vi "App - analyze RUS V6.vi"() -> ()   [LabVIEW 2021] (continued)
 "temperature str"="14.44900", "file path"=path "D:/Data/Ultrasound/LSCO/LSCO22__130814c/5_Cooling_2nd_try/September_2014/091814/14.44900K_500_2500_2.10000V_0.00000T_Sep18-2014__02-05-45_001_091814.bin", "last mod"=timestamp(3493865145 s since 1904-01-01), "file name str"="D:\\Data\\Ultrasound\\LSCO\\LSCO22__130814c\\5_Cooling_2nd_try\\September_2014\\091814\\14.44900K_500_2500_2.10000V_0.00000T_Sep18-2014__02-05-45_001_091814.bin", "mod time(min)"=58231085.75, "file format"=enum."binary", "power(V)"=2.1, "Magn Field(T) "=0.0}, {"temperature"=14.445, "temperature str"="14.44500", "file path"=path "D:/Data/Ultrasound/LSCO/LSCO22__130814c/5_Cooling_2nd_try/September_2014/091814/14.44500K_500_2500_2.10000V_0.00000T_Sep18-2014__02-07-04_001_091814.bin", "last mod"=timestamp(3493865224 s since 1904-01-01), "file name str"="D:\\Data\\Ultrasound\\LSCO\\LSCO22__130814c\\5_Cooling_2nd_try\\September_2014\\091814\\14.44500K_500_2500_2.10000V_0.00000T_Sep18-2014__02-07-04_001_091814.bin", "mod time(min)"=58231087.06666667, "file format"=enum."binary", "power(V)"=2.1, "Magn Field(T) "=0.0}, {"temperature"=14.447, "temperature str"="14.44700", "file path"=path "D:/Data/Ultrasound/LSCO/LSCO22__130814c/5_Cooling_2nd_try/September_2014/091814/14.44700K_500_2500_2.10000V_0.00000T_Sep18-2014__02-08-23_001_091814.bin", "last mod"=timestamp(3493865303 s since 1904-01-01), "file name str"="D:\\Data\\Ultrasound\\LSCO\\LSCO22__130814c\\5_Cooling_2nd_try\\September_2014\\091814\\14.44700K_500_2500_2.10000V_0.00000T_Sep18-2014__02-08-23_001_091814.bin", "mod time(min)"=58231088.38333333, "file format"=enum."binary", "power(V)"=2.1, "Magn Field(T) "=0.0}, {"temperature"=14.443, "temperature str"="14.44300", "file path"=path "D:/Data/Ultrasound/LSCO/LSCO22__130814c/5_Cooling_2nd_try/September_2014/091814/14.44300K_500_2500_2.10000V_0.00000T_Sep18-2014__02-09-43_001_091814.bin", "last mod"=timestamp(3493865383 s since 1904-01-01), "file name str"="D:\\Data\\Ultrasound\\LSCO\\LSCO22__130814c\\5_Cooling_2nd_try\\September_2014\\091814\\14.44300K_500_2500_2.10000V_0.00000T_Sep18-2014__02-09-43_001_091814.bin", "mod time(min)"=58231089.71666667, "file format"=enum."binary", "power(V)"=2.1, "Magn Field(T) "=0.0}, {"temperature"=14.439, "temperature str"="14.43900", "file path"=path "D:/Data/Ultrasound/LSCO/LSCO22__130814c/5_Cooling_2nd_try/September_2014/091814/14.43900K_500_2500_2.10000V_0.00000T_Sep18-2014__02-11-02_001_091814.bin", "last mod"=timestamp(3493865462 s since 1904-01-01), "file name str"="D:\\Data\\Ultrasound\\LSCO\\LSCO22__130814c\\5_Cooling_2nd_try\\September_2014\\091814\\14.43900K_500_2500_2.10000V_0.00000T_Sep18-2014__02-11-02_001_091814.bin", "mod time(min)"=58231091.03333333, "file format"=enum."binary", "power(V)"=2.1, "Magn Field(T) "=0.0}, {"temperature"=14.439, "temperature str"="14.43900", "file path"=path "D:/Data/Ultrasound/LSCO/LSCO22__130814c/5_Cooling_2nd_try/September_2014/091814/14.43900K_500_2500_2.10000V_0.00000T_Sep18-2014__02-12-21_001_091814.bin", "last mod"=timestamp(3493865541 s since 1904-01-01), "file name str"="D:\\Data\\Ultrasound\\LSCO\\LSCO22__130814c\\5_Cooling_2nd_try\\September_2014\\091814\\14.43900K_500_2500_2.10000V_0.00000T_Sep18-2014__02-12-21_001_091814.bin", "mod time(min)"=58231092.35, "file format"=enum."binary", "power(V)"=2.1, "Magn Field(T) "=0.0}, {"temperature"=14.439, "temperature str"="14.43900", "file path"=path "D:/Data/Ultrasound/LSCO/LSCO22__130814c/5_Cooling_2nd_try/September_2014/091814/14.43900K_500_2500_2.10000V_0.00000T_Sep18-2014__02-13-41_001_091814.bin", "last mod"=timestamp(3493865621 s since 1904-01-01), "file name str"="D:\\Data\\Ultrasound\\LSCO\\LSCO22__130814c\\5_Cooling_2nd_try\\September_2014\\091814\\14.43900K_500_2500_2.10000V_0.00000T_Sep18-2014__02-13-41_001_091814.bin", "mod time(min)"=58231093.68333333, "file format"=enum."binary", "power(V)"=2.1, "Magn Field(T) "=0.0}, {"temperature"=14.439, "temperature str"="14.43900", "file path"=path "D:/Data/Ultrasound/LSCO/LSCO22__130814c/5_Cooling_2nd_try/September_2014/091814/14.43900K_500_2500_2.10000V_0.00000T_Sep18-2014__02-15-00_001_091814.bin", "last mod"=timestamp(3493865700 s since 1904-01-01), "file name str"="D:\\Data\\Ultrasound\\LSCO\\LSCO22__130814c\\5_Cooling_2nd_try\\September_2014\\091814\\14.43900K_500_2500_2.10000V_0.00000T_Sep18-2014__02-15-00_001_091814.bin", "mod time(min)"=58231095.0, "file format"=enum."binary", "power(V)"=2.1, "Magn Field(T) "=0.0}, {"temperature"=14.44, "temperature str"="14.44000", "file path"=path "D:/Data/Ultrasound/LSCO/LSCO22__130814c/5_Cooling_2nd_try/September_2014/091814/14.44000K_500_2500_2.10000V_0.00000T_Sep18-2014__02-16-20_001_091814.bin", "last mod"=timestamp(3493865780 s since 1904-01-01), "file name str"="D:\\Data\\Ultrasound\\LSCO\\LSCO22__130814c\\5_Cooling_2nd_try\\September_2014\\091814\\14.44000K_500_2500_2.10000V_0.00000T_Sep18-2014__02-16-20_001_091814.bin", "mod time(min)"=58231096.333333336, "file format"=enum."binary", "power(V)"=2.1, "Magn Field(T) "=0.0}, {"temperature"=14.433, "temperature str"="14.43300", "file path"=path "D:/Data/Ultrasound/LSCO/LSCO22__130814c/5_Cooling_2nd_try/September_2014/091814/14.43300K_500_2500_2.10000V_0.00000T_Sep18-2014__02-17-39_001_091814.bin", "last mod"=timestamp(3493865859 s since 1904-01-01), "file name str"="D:\\Data\\Ultrasound\\LSCO\\LSCO22__130814c\\5_Cooling_2nd_try\\September_2014\\091814\\14.43300K_500_2500_2.10000V_0.00000T_Sep18-2014__02-17-39_001_091814.bin", "mod time(min)"=58231097.65, "file format"=enum."binary", "power(V)"=2.1, "Magn Field(T) "=0.0}, {"temperature"=14.434, "temperature str"="14.43400", "file path"=path "D:/Data/Ultrasound/LSCO/LSCO22__130814c/5_Cooling_2nd_try/September_2014/091814/14.43400K_500_2500_2.10000V_0.00000T_Sep18-2014__02-18-58_001_091814.bin", "last mod"=timestamp(3493865938 s since 1904-01-01), "file name str"="D:\\Data\\Ultrasound\\LSCO\\LSCO22__130814c\\5_Cooling_2nd_try\\September_2014\\091814\\14.43400K_500_2500_2.10000V_0.00000T_Sep18-2014__02-18-58_001_091814.bin", "mod time(min)"=58231098.96666667, "file format"=enum."binary", "power(V)"=2.1, "Magn Field(T) "=0.0}, {"temperature"=14.43, "temperature str"="14.43000", "file path"=path "D:/Data/Ultrasound/LSCO/LSCO22__130814c/5_Cooling_2nd_try/September_2014/091814/14.43000K_500_2500_2.10000V_0.00000T_Sep18-2014__02-20-18_001_091814.bin", "last mod"=timestamp(3493866018 s since 1904-01-01), "file name str"="D:\\Data\\Ultrasound\\LSCO\\LSCO22__130814c\\5_Cooling_2nd_try\\September_2014\\091814\\14.43000K_500_2500_2.10000V_0.00000T_Sep18-2014__02-20-18_001_091814.bin", "mod time(min)"=58231100.3, "file format"=enum."binary", "power(V)"=2.1, "Magn Field(T) "=0.0}, {"temperature"=14.43, "temperature str"="14.43000", "file path"=path "D:/Data/Ultrasound/LSCO/LSCO22__130814c/5_Cooling_2nd_try/September_2014/091814/14.43000K_500_2500_2.10000V_0.00000T_Sep18-2014__02-21-37_001_091814.bin", "last mod"=timestamp(3493866097 s since 1904-01-01), "file name str"="D:\\Data\\Ultrasound\\LSCO\\LSCO22__130814c\\5_Cooling_2nd_try\\September_2014\\091814\\14.43000K_500_2500_2.10000V_0.00000T_Sep18-2014__02-21-37_001_091814.bin", "mod time(min)"=58231101.61666667, "file format"=enum."binary", "power(V)"=2.1, "Magn Field(T) "=0.0}, {"temperature"=14.43, "temperature str"="14.43000", "file path"=path "D:/Data/Ultrasound/LSCO/LSCO22__130814c/5_Cooling_2nd_try/September_2014/091814/14.43000K_500_2500_2.10000V_0.00000T_Sep18-2014__02-22-57_001_091814.bin", "last mod"=timestamp(3493866177 s since 1904-01-01), "file name str"="D:\\Data\\Ultrasound\\LSCO\\LSCO22__130814c\\5_Cooling_2nd_try\\September_2014\\091814\\14.43000K_500_2500_2.10000V_0.00000T_Sep18-2014__02-22-57_001_091814.bin", "mod time(min)"=58231102.95, "file format"=enum."binary", "power(V)"=2.1, "Magn Field(T) "=0.0}, {"temperature"=14.434, "temperature str"="14.43400", "file path"=path "D:/Data/Ultrasound/LSCO/LSCO22__130814c/5_Cooling_2nd_try/September_2014/091814/14.43400K_500_2500_2.10000V_0.00000T_Sep18-2014__02-24-16_001_091814.bin", "last mod"=timestamp(3493866256 s since 1904-01-01), "file name str"="D:\\Data\\Ultrasound\\LSCO\\LSCO22__130814c\\5_Cooling_2nd_try\\September_2014\\091814\\14.43400K_500_2500_2.10000V_0.00000T_Sep18-2014__02-24-16_001_091814.bin", "mod time(min)"=58231104.266666666, "file format"=enum."binary", "power(V)"=2.1, "Magn Field(T) "=0.0}, {"temperature"=14.434, "temperature str"="14.43400", "file path"=path "D:/Data/Ultrasound/LSCO/LSCO22__130814c/5_Cooling_2nd_try/September_2014/091814/14.43400K_500_2500_2.10000V_0.00000T_Sep18-2014__02-25-35_001_091814.bin", "last mod"=timestamp(3493866335 s since 1904-01-01), "file name str"="D:\\Data\\Ultrasound\\LSCO\\LSCO22__130814c\\5_Cooling_2nd_try\\September_2014\\091814\\14.43400K_500_2500_2.10000V_0.00000T_Sep18-2014__02-25-35_001_091814.bin", "mod time(min)"=58231105.583333336, "file format"=enum."binary", "power(V)"=2.1, "Magn Field(T) "=0.0}, {"temperature"=14.431, "temperature str"="14.43100", "file path"=path "D:/Data/Ultrasound/LSCO/LSCO22__130814c/5_Cooling_2nd_try/September_2014/091814/14.43100K_500_2500_2.10000V_0.00000T_Sep18-2014__02-26-55_001_091814.bin", "last mod"=timestamp(3493866415 s since 1904-01-01), "file name str"="D:\\Data\\Ultrasound\\LSCO\\LSCO22__130814c\\5_Cooling_2nd_try\\September_2014\\091814\\14.43100K_500_2500_2.10000V_0.00000T_Sep18-2014__02-26-55_001_091814.bin", "mod time(min)"=58231106.916666664, "file format"=enum."binary", "power(V)"=2.1, "Magn Field(T) "=0.0}, {"temperature"=14.429, "temperature str"="14.42900", "file path"=path "D:/Data/Ultrasound/LSCO/LSCO22__130814c/5_Cooling_2nd_try/September_2014/091814/14.42900K_500_2500_2.10000V_0.00000T_Sep18-2014__02-28-14_001_091814.bin", "last mod"=timestamp(3493866494 s since 1904-01-01), "file name str"="D:\\Data\\Ultrasound\\LSCO\\LSCO22__130814c\\5_Cooling_2nd_try\\September_2014\\091814\\14.42900K_500_2500_2.10000V_0.00000T_Sep18-2014__02-28-14_001_091814.bin", "mod time(min)"=58231108.233333334, "file format"=enum."binary", "power(V)"=2.1, "Magn Field(T) "=0.0}, {"temperature"=14.426, "temperature str"="14.42600", "file path"=path "D:/Data/Ultrasound/LSCO/LSCO22__130814c/5_Cooling_2nd_try/September_2014/091814/14.42600K_500_2500_2.10000V_0.00000T_Sep18-2014__02-29-33_001_091814.bin", "last mod"=timestamp(3493866573 s since 1904-01-01), "file name str"="D:\\Data\\Ultrasound\\LSCO\\LSCO22__130814c\\5_Cooling_2nd_try\\September_2014\\091814\\14.42600K_500_2500_2.10000V_0.00000T_Sep18-2014__02-29-33_001_091814.bin", "mod time(min)"=58231109.55, "file format"=enum."binary", "power(V)"=2.1, "Magn Field(T) "=0.0}, {"temperature"=14.429, "temperature str"="14.42900", "file path"=path "D:/Data/Ultrasound/LSCO/LSCO22__130814c/5_Cooling_2nd_try/September_2014/091814/14.42900K_500_2500_2.10000V_0.00000T_Sep18-2014__02-30-53_001_091814.bin", "last mod"=timestamp(3493866653 s since 1904-01-01), "file name str"="D:\\Data\\Ultrasound\\LSCO\\LSCO22__130814c\\5_Cooling_2nd_try\\September_2014\\091814\\14.42900K_500_2500_2.10000V_0.00000T_Sep18-2014__02-30-53_001_091814.bin", "mod time(min)"=58231110.88333333, "file format"=enum."binary", "power(V)"=2.1, "Magn Field(T) "=0.0}, {"temperature"=14.429, "temperature str"="14.42900", "file path"=path "D:/Data/Ultrasound/LSCO/LSCO22__130814c/5_Cooling_2nd_try/September_2014/091814/14.42900K_500_2500_2.10000V_0.00000T_Sep18-2014__02-32-12_001_091814.bin", "last mod"=timestamp(3493866732 s since 1904-01-01), "file name str"="D:\\Data\\Ultrasound\\LSCO\\LSCO22__130814c\\5_Cooling_2nd_try\\September_2014\\091814\\14.42900K_500_2500_2.10000V_0.00000T_Sep18-2014__02-32-12_001_091814.bin", "mod time(min)"=58231112.2, "file format"=enum."binary", "power(V)"=2.1, "Magn Field(T) "=0.0}, {"temperature"=14.425, "temperature str"="14.42500", "file path"=path "D:/Data/Ultrasound/LSCO/LSCO22__130814c/5_Cooling_2nd_try/September_2014/091814/14.42500K_500_2500_2.10000V_0.00000T_Sep18-2014__02-33-32_001_091814.bin", "last mod"=timestamp(3493866812 s since 1904-01-01), "file name str"="D:\\Data\\Ultrasound\\LSCO\\LSCO22__130814c\\5_Cooling_2nd_try\\September_2014\\091814\\14.42500K_500_2500_2.10000V_0.00000T_Sep18-2014__02-33-32_001_091814.bin", "mod time(min)"=58231113.53333333, "file format"=enum."binary", "power(V)"=2.1, "Magn Field(T) "=0.0}, {"temperature"=14.426, "temperature str"="14.42600", "file path"=path "D:/Data/Ultrasound/LSCO/LSCO22__130814c/5_Cooling_2nd_try/September_2014/091814/14.42600K_500_2500_2.10000V_0.00000T_Sep18-2014__02-34-51_001_091814.bin", "last mod"=timestamp(3493866891 s since 1904-01-01), "file name str"="D:\\Data\\Ultrasound\\LSCO\\LSCO22__130814c\\5_Cooling_2nd_try\\September_2014\\091814\\14.42600K_500_2500_2.10000V_0.00000T_Sep18-2014__02-34-51_001_091814.bin", "mod time(min)"=58231114.85, "file format"=enum."binary", "power(V)"=2.1, "Magn Field(T) "=0.0}, {"temperature"=14.422, "temperature str"="14.42200", "file path"=path "D:/Data/Ultrasound/LSCO/LSCO22__130814c/5_Cooling_2nd_try/September_2014/091814/14.42200K_500_2500_2.10000V_0.00000T_Sep18-2014__02-36-10_001_091814.bin", "last mod"=timestamp(3493866970 s since 1904-01-01), "file name str"="D:\\Data\\Ultrasound\\LSCO\\LSCO22__130814c\\5_Cooling_2nd_try\\September_2014\\091814\\14.42200K_500_2500_2.10000V_0.00000T_Sep18-2014__02-36-10_001_091814.bin", "mod time(min)"=58231116.166666664, "file format"=enum."binary", "power(V)"=2.1, "Magn Field(T) "=0.0}, {"temperature"=14.424, "temperature str"="14.42400", "file path"=path "D:/Data/Ultrasound/LSCO/LSCO22__130814c/5_Cooling_2nd_try/September_2014/091814/14.42400K_500_2500_2.10000V_0.00000T_Sep18-2014__02-37-30_001_091814.bin", "last mod"=timestamp(3493867050 s since 1904-01-01), "file name str"="D:\\Data\\Ultrasound\\LSCO\\LSCO22__130814c\\5_Cooling_2nd_try\\September_2014\\091814\\14.42400K_500_2500_2.10000V_0.00000T_Sep18-2014__02-37-30_001_091814.bin", "mod time(min)"=58231117.5, "file format"=enum."binary", "power(V)"=2.1, "Magn Field(T) "=0.0}, {"temperature"=14.421, "temperature str"="14.42100", "file path"=path "D:/Data/Ultrasound/LSCO/LSCO22__130814c/5_Cooling_2nd_try/September_2014/091814/14.42100K_500_2500_2.10000V_0.00000T_Sep18-2014__02-38-49_001_091814.bin", "last mod"=timestamp(3493867129 s since 1904-01-01), "file name str"="D:\\Data\\Ultrasound\\LSCO\\LSCO22__130814c\\5_Cooling_2nd_try\\September_2014\\091814\\14.42100K_500_2500_2.10000V_0.00000T_Sep18-2014__02-38-49_001_091814.bin", "mod time(min)"=58231118.81666667, "file format"=enum."binary", "power(V)"=2.1, "Magn Field(T) "=0.0}, {"temperature"=14.418, "temperature str"="14.41800", "file path"=path "D:/Data/Ultrasound/LSCO/LSCO22__130814c/5_Cooling_2nd_try/September_2014/091814/14.41800K_500_2500_2.10000V_0.00000T_Sep18-2014__02-40-08_001_091814.bin", "last mod"=timestamp(3493867208 s since 1904-01-01), "file name str"="D:\\Data\\Ultrasound\\LSCO\\LSCO22__130814c\\5_Cooling_2nd_try\\September_2014\\091814\\14.41800K_500_2500_2.10000V_0.00000T_Sep18-2014__02-40-08_001_091814.bin", "mod time(min)"=58231120.13333333, "file format"=enum."binary", "power(V)"=2.1, "Magn Field(T) "=0.0}, {"temperature"=14.417, "temperature str"="14.41700", "file path"=path "D:/Data/Ultrasound/LSCO/LSCO22__130814c/5_Cooling_2nd_try/September_2014/091814/14.41700K_500_2500_2.10000V_0.00000T_Sep18-2014__02-41-28_001_091814.bin", "last mod"=timestamp(3493867288 s since 1904-01-01), "file name str"="D:\\Data\\Ultrasound\\LSCO\\LSCO22__130814c\\5_Cooling_2nd_try\\September_2014\\091814\\14.41700K_500_2500_2.10000V_0.00000T_Sep18-2014__02-41-28_001_091814.bin", "mod time(min)"=58231121.46666667, "file format"=enum."binary", "power(V)"=2.1, "Magn Field(T) "=0.0}, {"temperature"=14.415, "temperature str"="14.41500", "file path"=path "D:/Data/Ultrasound/LSCO/LSCO22__130814c/5_Cooling_2nd_try/September_2014/091814/14.41500K_500_2500_2.10000V_0.00000T_Sep18-2014__02-42-47_001_091814.bin", "last mod"=timestamp(3493867367 s since 1904-01-01), "file name str"="D:\\Data\\Ultrasound\\LSCO\\LSCO22__130814c\\5_Cooling_2nd_try\\September_2014\\091814\\14.41500K_500_2500_2.10000V_0.00000T_Sep18-2014__02-42-47_001_091814.bin", "mod time(min)"=58231122.78333333, "file format"=enum."binary", "power(V)"=2.1, "Magn Field(T) "=0.0}, {"temperature"=14.413, "temperature str"="14.41300", "file path"=path "D:/Data/Ultrasound/LSCO/LSCO22__130814c/5_Cooling_2nd_try/September_2014/091814/14.41300K_500_2500_2.10000V_0.00000T_Sep18-2014__02-44-07_001_091814.bin", "last mod"=timestamp(3493867447 s since 1904-01-01), "file name str"="D:\\Data\\Ultrasound\\LSCO\\LSCO22__130814c\\5_Cooling_2nd_try\\September_2014\\091814\\14.41300K_500_2500_2.10000V_0.00000T_Sep18-2014__02-44-07_001_091814.bin", "mod time(min)"=58231124.11666667, "file format"=enum."binary", "power(V)"=2.1, "Magn Field(T) "=0.0}, {"temperature"=14.414, "temperature str"="14.41400", "file path"=path "D:/Data/Ultrasound/LSCO/LSCO22__130814c/5_Cooling_2nd_try/September_2014/091814/14.41400K_500_2500_2.10000V_0.00000T_Sep18-2014__02-45-26_001_091814.bin", "last mod"=timestamp(3493867526 s since 1904-01-01), "file name str"="D:\\Data\\Ultrasound\\LSCO\\LSCO22__130814c\\5_Cooling_2nd_try\\September_2014\\091814\\14.41400K_500_2500_2.10000V_0.00000T_Sep18-2014__02-45-26_001_091814.bin", "mod time(min)"=58231125.43333333, "file format"=enum."binary", "power(V)"=2.1, "Magn Field(T) "=0.0}, {"temperature"=14.412, "temperature str"="14.41200", "file path"=path "D:/Data/Ultrasound/LSCO/LSCO22__130814c/5_Cooling_2nd_try/September_2014/091814/14.41200K_500_2500_2.10000V_0.00000T_Sep18-2014__02-46-45_001_091814.bin", "last mod"=timestamp(3493867605 s since 1904-01-01), "file name str"="D:\\Data\\Ultrasound\\LSCO\\LSCO22__130814c\\5_Cooling_2nd_try\\September_2014\\091814\\14.41200K_500_2500_2.10000V_0.00000T_Sep18-2014__02-46-45_001_091814.bin", "mod time(min)"=58231126.75, "file format"=enum."binary", "power(V)"=2.1, "Magn Field(T) "=0.0}, {"temperature"=14.418, "temperature str"="14.41800", "file path"=path "D:/Data/Ultrasound/LSCO/LSCO22__130814c/5_Cooling_2nd_try/September_2014/091814/14.41800K_500_2500_2.10000V_0.00000T_Sep18-2014__02-48-05_001_091814.bin", "last mod"=timestamp(3493867685 s since 1904-01-01), "file name str"="D:\\Data\\Ultrasound\\LSCO\\LSCO22__130814c\\5_Cooling_2nd_try\\September_2014\\091814\\14.41800K_500_2500_2.10000V_0.00000T_Sep18-2014__02-48-05_001_091814.bin", "mod time(min)"=58231128.083333336, "file format"=enum."binary", "power(V)"=2.1, "Magn Field(T) "=0.0}, {"temperature"=14.417, "temperature str"="14.41700", "file path"=path "D:/Data/Ultrasound/LSCO/LSCO22__130814c/5_Cooling_2nd_try/September_2014/091814/14.41700K_500_2500_2.10000V_0.00000T_Sep18-2014__02-49-24_001_091814.bin", "last mod"=timestamp(3493867764 s since 1904-01-01), "file name str"="D:\\Data\\Ultrasound\\LSCO\\LSCO22__130814c\\5_Cooling_2nd_try\\September_2014\\091814\\14.41700K_500_2500_2.10000V_0.00000T_Sep18-2014__02-49-24_001_091814.bin", "mod time(min)"=58231129.4, "file format"=enum."binary", "power(V)"=2.1, "Magn Field(T) "=0.0}, {"temperature"=14.412, "temperature str"="14.41200", "file path"=path "D:/Data/Ultrasound/LSCO/LSCO22__130814c/5_Cooling_2nd_try/September_2014/091814/14.41200K_500_2500_2.10000V_0.00000T_Sep18-2014__02-50-44_001_091814.bin", "last mod"=timestamp(3493867844 s since 1904-01-01), "file name str"="D:\\Data\\Ultrasound\\LSCO\\LSCO22__130814c\\5_Cooling_2nd_try\\September_2014\\091814\\14.41200K_500_2500_2.10000V_0.00000T_Sep18-2014__02-50-44_001_091814.bin", "mod time(min)"=58231130.733333334, "file format"=enum."binary", "power(V)"=2.1, "Magn Field(T) "=0.0}, {"temperature"=14.413, "temperature str"="14.41300", "file path"=path "D:/Data/Ultrasound/LSCO/LSCO22__130814c/5_Cooling_2nd_try/September_2014/091814/14.41300K_500_2500_2.10000V_0.00000T_Sep18-2014__02-52-03_001_091814.bin", "last mod"=timestamp(3493867923 s since 1904-01-01), "file name str"="D:\\Data\\Ultrasound\\LSCO\\LSCO22__130814c\\5_Cooling_2nd_try\\September_2014\\091814\\14.41300K_500_2500_2.10000V_0.00000T_Sep18-2014__02-52-03_001_091814.bin", "mod time(min)"=58231132.05, "file format"=enum."binary", "power(V)"=2.1, "Magn Field(T) "=0.0}, {"temperature"=14.41, "temperature str"="14.41000", "file path"=path "D:/Data/Ultrasound/LSCO/LSCO22__130814c/5_Cooling_2nd_try/September_2014/091814/14.41000K_500_2500_2.10000V_0.00000T_Sep18-2014__02-53-22_001_091814.bin", "last mod"=timestamp(3493868002 s since 1904-01-01), "file name str"="D:\\Data\\Ultrasound\\LSCO\\LSCO22__130814c\\5_Cooling_2nd_try\\September_2014\\091814\\14.41000K_500_2500_2.10000V_0.00000T_Sep18-2014__02-53-22_001_091814.bin", "mod time(min)"=58231133.36666667, "file format"=enum."binary", "power(V)"=2.1, "Magn Field(T) "=0.0}, {"temperature"=14.414, "temperature str"="14.41400", "file path"=path "D:/Data/Ultrasound/LSCO/LSCO22__130814c/5_Cooling_2nd_try/September_2014/091814/14.41400K_500_2500_2.10000V_0.00000T_Sep18-2014__02-54-42_001_091814.bin", "last mod"=timestamp(3493868082 s since 1904-01-01), "file name str"="D:\\Data\\Ultrasound\\LSCO\\LSCO22__130814c\\5_Cooling_2nd_try\\September_2014\\091814\\14.41400K_500_2500_2.10000V_0.00000T_Sep18-2014__02-54-42_001_091814.bin", "mod time(min)"=58231134.7, "file format"=enum."binary", "power(V)"=2.1, "Magn Field(T) "=0.0}, {"temperature"=14.408, "temperature str"="14.40800", "file path"=path "D:/Data/Ultrasound/LSCO/LSCO22__130814c/5_Cooling_2nd_try/September_2014/091814/14.40800K_500_2500_2.10000V_0.00000T_Sep18-2014__02-56-01_001_091814.bin", "last mod"=timestamp(3493868161 s since 1904-01-01), "file name str"="D:\\Data\\Ultrasound\\LSCO\\LSCO22__130814c\\5_Cooling_2nd_try\\September_2014\\091814\\14.40800K_500_2500_2.10000V_0.00000T_Sep18-2014__02-56-01_001_091814.bin", "mod time(min)"=58231136.016666666, "file format"=enum."binary", "power(V)"=2.1, "Magn Field(T) "=0.0}, {"temperature"=14.407, "temperature str"="14.40700", "file path"=path "D:/Data/Ultrasound/LSCO/LSCO22__130814c/5_Cooling_2nd_try/September_2014/091814/14.40700K_500_2500_2.10000V_0.00000T_Sep18-2014__02-57-20_001_091814.bin", "last mod"=timestamp(3493868240 s since 1904-01-01), "file name str"="D:\\Data\\Ultrasound\\LSCO\\LSCO22__130814c\\5_Cooling_2nd_try\\September_2014\\091814\\14.40700K_500_2500_2.10000V_0.00000T_Sep18-2014__02-57-20_001_091814.bin", "mod time(min)"=58231137.333333336, "file format"=enum."binary", "power(V)"=2.1, "Magn Field(T) "=0.0}, {"temperature"=14.406, "temperature str"="14.40600", "file path"=path "D:/Data/Ultrasound/LSCO/LSCO22__130814c/5_Cooling_2nd_try/September_2014/091814/14.40600K_500_2500_2.10000V_0.00000T_Sep18-2014__02-58-40_001_091814.bin", "last mod"=timestamp(3493868320 s since 1904-01-01), "file name str"="D:\\Data\\Ultrasound\\LSCO\\LSCO22__130814c\\5_Cooling_2nd_try\\September_2014\\091814\\14.40600K_500_2500_2.10000V_0.00000T_Sep18-2014__02-58-40_001_091814.bin", "mod time(min)"=58231138.666666664, "file format"=enum."binary", "power(V)"=2.1, "Magn Field(T) "=0.0}, {"temperature"=14.402, "temperature str"="14.40200", "file path"=path "D:/Data/Ultrasound/LSCO/LSCO22__130814c/5_Cooling_2nd_try/September_2014/091814/14.40200K_500_2500_2.10000V_0.00000T_Sep18-2014__02-59-59_001_091814.bin", "last mod"=timestamp(3493868399 s since 1904-01-01), "file name str"="D:\\Data\\Ultrasound\\LSCO\\LSCO22__130814c\\5_Cooling_2nd_try\\September_2014\\091814\\14.40200K_500_2500_2.10000V_0.00000T_Sep18-2014__02-59-59_001_091814.bin", "mod time(min)"=58231139.983333334, "file format"=enum."binary", "power(V)"=2.1, "Magn Field(T) "=0.0}, {"temperature"=14.4, "temperature str"="14.40000", "file path"=path "D:/Data/Ultrasound/LSCO/LSCO22__130814c/5_Cooling_2nd_try/September_2014/091814/14.40000K_500_2500_2.10000V_0.00000T_Sep18-2014__03-01-19_001_091814.bin", "last mod"=timestamp(3493868479 s since 1904-01-01), "file name str"="D:\\Data\\Ultrasound\\LSCO\\LSCO22__130814c\\5_Cooling_2nd_try\\September_2014\\091814\\14.40000K_500_2500_2.10000V_0.00000T_Sep18-2014__03-01-19_001_091814.bin", "mod time(min)"=58231141.31666667, "file format"=enum."binary", "power(V)"=2.1, "Magn Field(T) "=0.0}, {"temperature"=14.396, "temperature str"="14.39600", "file path"=path "D:/Data/Ultrasound/LSCO/LSCO22__130814c/5_Cooling_2nd_try/September_2014/091814/14.39600K_500_2500_2.10000V_0.00000T_Sep18-2014__03-02-38_001_091814.bin", "last mod"=timestamp(3493868558 s since 1904-01-01), "file name str"="D:\\Data\\Ultrasound\\LSCO\\LSCO22__130814c\\5_Cooling_2nd_try\\September_2014\\091814\\14.39600K_500_2500_2.10000V_0.00000T_Sep18-2014__03-02-38_001_091814.bin", "mod time(min)"=58231142.63333333, "file format"=enum."binary", "power(V)"=2.1, "Magn Field(T) "=0.0}, {"temperature"=14.394, "temperature str"="14.39400", "file path"=path "D:/Data/Ultrasound/LSCO/LSCO22__130814c/5_Cooling_2nd_try/September_2014/091814/14.39400K_500_2500_2.10000V_0.00000T_Sep18-2014__03-03-57_001_091814.bin", "last mod"=timestamp(3493868637 s since 1904-01-01), "file name str"="D:\\Data\\Ultrasound\\LSCO\\LSCO22__130814c\\5_Cooling_2nd_try\\September_2014\\091814\\14.39400K_500_2500_2.10000V_0.00000T_Sep18-2014__03-03-57_001_091814.bin", "mod time(min)"=58231143.95, "file format"=enum."binary", "power(V)"=2.1, "Magn Field(T) "=0.0}, {"temperature"=14.393, "temperature str"="14.39300", "file path"=path "D:/Data/Ultrasound/LSCO/LSCO22__130814c/5_Cooling_2nd_try/September_2014/091814/14.39300K_500_2500_2.10000V_0.00000T_Sep18-2014__03-05-17_001_091814.bin", "last mod"=timestamp(3493868717 s since 1904-01-01), "file name str"="D:\\Data\\Ultrasound\\LSCO\\LSCO22__130814c\\5_Cooling_2nd_try\\September_2014\\091814\\14.39300K_500_2500_2.10000V_0.00000T_Sep18-2014__03-05-17_001_091814.bin", "mod time(min)"=58231145.28333333, "file format"=enum."binary", "power(V)"=2.1, "Magn Field(T) "=0.0}, {"temperature"=14.39, "temperature str"="14.39000", "file path"=path "D:/Data/Ultrasound/LSCO/LSCO22__130814c/5_Cooling_2nd_try/September_2014/091814/14.39000K_500_2500_2.10000V_0.00000T_Sep18-2014__03-06-36_001_091814.bin", "last mod"=timestamp(3493868796 s since 1904-01-01), "file name str"="D:\\Data\\Ultrasound\\LSCO\\LSCO22__130814c\\5_Cooling_2nd_try\\September_2014\\091814\\14.39000K_500_2500_2.10000V_0.00000T_Sep18-2014__03-06-36_001_091814.bin", "mod time(min)"=58231146.6, "file format"=enum."binary", "power(V)"=2.1, "Magn Field(T) "=0.0}, {"temperature"=14.387, "temperature str"="14.38700", "file path"=path "D:/Data/Ultrasound/LSCO/LSCO22__130814c/5_Cooling_2nd_try/September_2014/091814/14.38700K_500_2500_2.10000V_0.00000T_Sep18-2014__03-07-56_001_091814.bin", "last mod"=timestamp(3493868876 s since 1904-01-01), "file name str"="D:\\Data\\Ultrasound\\LSCO\\LSCO22__130814c\\5_Cooling_2nd_try\\September_2014\\091814\\14.38700K_500_2500_2.10000V_0.00000T_Sep18-2014__03-07-56_001_091814.bin", "mod time(min)"=58231147.93333333, "file format"=enum."binary", "power(V)"=2.1, "Magn Field(T) "=0.0}, {"temperature"=14.39, "temperature str"="14.39000", "file path"=path "D:/Data/Ultrasound/LSCO/LSCO22__130814c/5_Cooling_2nd_try/September_2014/091814/14.39000K_500_2500_2.10000V_0.00000T_Sep18-2014__03-09-15_001_091814.bin", "last mod"=timestamp(3493868955 s since 1904-01-01), "file name str"="D:\\Data\\Ultrasound\\LSCO\\LSCO22__130814c\\5_Cooling_2nd_try\\September_2014\\091814\\14.39000K_500_2500_2.10000V_0.00000T_Sep18-2014__03-09-15_001_091814.bin", "mod time(min)"=58231149.25, "file format"=enum."binary", "power(V)"=2.1, "Magn Field(T) "=0.0}, {"temperature"=14.385, "temperature str"="14.38500", "file path"=path "D:/Data/Ultrasound/LSCO/LSCO22__130814c/5_Cooling_2nd_try/September_2014/091814/14.38500K_500_2500_2.10000V_0.00000T_Sep18-2014__03-10-34_001_091814.bin", "last mod"=timestamp(3493869034 s since 1904-01-01), "file name str"="D:\\Data\\Ultrasound\\LSCO\\LSCO22__130814c\\5_Cooling_2nd_try\\September_2014\\091814\\14.38500K_500_2500_2.10000V_0.00000T_Sep18-2014__03-10-34_001_091814.bin", "mod time(min)"=58231150.56666667, "file format"=enum."binary", "power(V)"=2.1, "Magn Field(T) "=0.0}, {"temperature"=14.384, "temperature str"="14.38400", "file path"=path "D:/Data/Ultrasound/LSCO/LSCO22__130814c/5_Cooling_2nd_try/September_2014/091814/14.38400K_500_2500_2.10000V_0.00000T_Sep18-2014__03-11-54_001_091814.bin", "last mod"=timestamp(3493869114 s since 1904-01-01), "file name str"="D:\\Data\\Ultrasound\\LSCO\\LSCO22__130814c\\5_Cooling_2nd_try\\September_2014\\091814\\14.38400K_500_2500_2.10000V_0.00000T_Sep18-2014__03-11-54_001_091814.bin", "mod time(min)"=58231151.9, "file format"=enum."binary", "power(V)"=2.1, "Magn Field(T) "=0.0}, {"temperature"=14.387, "temperature str"="14.38700", "file path"=path "D:/Data/Ultrasound/LSCO/LSCO22__130814c/5_Cooling_2nd_try/September_2014/091814/14.38700K_500_2500_2.10000V_0.00000T_Sep18-2014__03-13-13_001_091814.bin", "last mod"=timestamp(3493869193 s since 1904-01-01), "file name str"="D:\\Data\\Ultrasound\\LSCO\\LSCO22__130814c\\5_Cooling_2nd_try\\September_2014\\091814\\14.38700K_500_2500_2.10000V_0.00000T_Sep18-2014__03-13-13_001_091814.bin", "mod time(min)"=58231153.21666667, "file format"=enum."binary", "power(V)"=2.1, "Magn Field(T) "=0.0}, {"temperature"=14.388, "temperature str"="14.38800", "file path"=path "D:/Data/Ultrasound/LSCO/LSCO22__130814c/5_Cooling_2nd_try/September_2014/091814/14.38800K_500_2500_2.10000V_0.00000T_Sep18-2014__03-14-32_001_091814.bin", "last mod"=timestamp(3493869272 s since 1904-01-01), "file name str"="D:\\Data\\Ultrasound\\LSCO\\LSCO22__130814c\\5_Cooling_2nd_try\\September_2014\\091814\\14.38800K_500_2500_2.10000V_0.00000T_Sep18-2014__03-14-32_001_091814.bin", "mod time(min)"=58231154.53333333, "file format"=enum."binary", "power(V)"=2.1, "Magn Field(T) "=0.0}, {"temperature"=14.382, "temperature str"="14.38200", "file path"=path "D:/Data/Ultrasound/LSCO/LSCO22__130814c/5_Cooling_2nd_try/September_2014/091814/14.38200K_500_2500_2.10000V_0.00000T_Sep18-2014__03-15-52_001_091814.bin", "last mod"=timestamp(3493869352 s since 1904-01-01), "file name str"="D:\\Data\\Ultrasound\\LSCO\\LSCO22__130814c\\5_Cooling_2nd_try\\September_2014\\091814\\14.38200K_500_2500_2.10000V_0.00000T_Sep18-2014__03-15-52_001_091814.bin", "mod time(min)"=58231155.86666667, "file format"=enum."binary", "power(V)"=2.1, "Magn Field(T) "=0.0}, {"temperature"=14.384, "temperature str"="14.38400", "file path"=path "D:/Data/Ultrasound/LSCO/LSCO22__130814c/5_Cooling_2nd_try/September_2014/091814/14.38400K_500_2500_2.10000V_0.00000T_Sep18-2014__03-17-11_001_091814.bin", "last mod"=timestamp(3493869431 s since 1904-01-01), "file name str"="D:\\Data\\Ultrasound\\LSCO\\LSCO22__130814c\\5_Cooling_2nd_try\\September_2014\\091814\\14.38400K_500_2500_2.10000V_0.00000T_Sep18-2014__03-17-11_001_091814.bin", "mod time(min)"=58231157.18333333, "file format"=enum."binary", "power(V)"=2.1, "Magn Field(T) "=0.0}, {"temperature"=14.381, "temperature str"="14.38100", "file path"=path "D:/Data/Ultrasound/LSCO/LSCO22__130814c/5_Cooling_2nd_try/September_2014/091814/14.38100K_500_2500_2.10000V_0.00000T_Sep18-2014__03-18-31_001_091814.bin", "last mod"=timestamp(3493869511 s since 1904-01-01), "file name str"="D:\\Data\\Ultrasound\\LSCO\\LSCO22__130814c\\5_Cooling_2nd_try\\September_2014\\091814\\14.38100K_500_2500_2.10000V_0.00000T_Sep18-2014__03-18-31_001_091814.bin", "mod time(min)"=58231158.516666666, "file format"=enum."binary", "power(V)"=2.1, "Magn Field(T) "=0.0}, {"temperature"=14.381, "temperature str"="14.38100", "file path"=path "D:/Data/Ultrasound/LSCO/LSCO22__130814c/5_Cooling_2nd_try/September_2014/091814/14.38100K_500_2500_2.10000V_0.00000T_Sep18-2014__03-19-50_001_091814.bin", "last mod"=timestamp(3493869590 s since 1904-01-01), "file name str"="D:\\Data\\Ultrasound\\LSCO\\LSCO22__130814c\\5_Cooling_2nd_try\\September_2014\\091814\\14.38100K_500_2500_2.10000V_0.00000T_Sep18-2014__03-19-50_001_091814.bin", "mod time(min)"=58231159.833333336, "file format"=enum."binary", "power(V)"=2.1, "Magn Field(T) "=0.0}, {"temperature"=14.376, "temperature str"="14.37600", "file path"=path "D:/Data/Ultrasound/LSCO/LSCO22__130814c/5_Cooling_2nd_try/September_2014/091814/14.37600K_500_2500_2.10000V_0.00000T_Sep18-2014__03-21-09_001_091814.bin", "last mod"=timestamp(3493869669 s since 1904-01-01), "file name str"="D:\\Data\\Ultrasound\\LSCO\\LSCO22__130814c\\5_Cooling_2nd_try\\September_2014\\091814\\14.37600K_500_2500_2.10000V_0.00000T_Sep18-2014__03-21-09_001_091814.bin", "mod time(min)"=58231161.15, "file format"=enum."binary", "power(V)"=2.1, "Magn Field(T) "=0.0}, {"temperature"=14.375, "temperature str"="14.37500", "file path"=path "D:/Data/Ultrasound/LSCO/LSCO22__130814c/5_Cooling_2nd_try/September_2014/091814/14.37500K_500_2500_2.10000V_0.00000T_Sep18-2014__03-22-29_001_091814.bin", "last mod"=timestamp(3493869749 s since 1904-01-01), "file name str"="D:\\Data\\Ultrasound\\LSCO\\LSCO22__130814c\\5_Cooling_2nd_try\\September_2014\\091814\\14.37500K_500_2500_2.10000V_0.00000T_Sep18-2014__03-22-29_001_091814.bin", "mod time(min)"=58231162.483333334, "file format"=enum."binary", "power(V)"=2.1, "Magn Field(T) "=0.0}, {"temperature"=14.371, "temperature str"="14.37100", "file path"=path "D:/Data/Ultrasound/LSCO/LSCO22__130814c/5_Cooling_2nd_try/September_2014/091814/14.37100K_500_2500_2.10000V_0.00000T_Sep18-2014__03-23-48_001_091814.bin", "last mod"=timestamp(3493869828 s since 1904-01-01), "file name str"="D:\\Data\\Ultrasound\\LSCO\\LSCO22__130814c\\5_Cooling_2nd_try\\September_2014\\091814\\14.37100K_500_2500_2.10000V_0.00000T_Sep18-2014__03-23-48_001_091814.bin", "mod time(min)"=58231163.8, "file format"=enum."binary", "power(V)"=2.1, "Magn Field(T) "=0.0}, {"temperature"=14.371, "temperature str"="14.37100", "file path"=path "D:/Data/Ultrasound/LSCO/LSCO22__130814c/5_Cooling_2nd_try/September_2014/091814/14.37100K_500_2500_2.10000V_0.00000T_Sep18-2014__03-25-07_001_091814.bin", "last mod"=timestamp(3493869907 s since 1904-01-01), "file name str"="D:\\Data\\Ultrasound\\LSCO\\LSCO22__130814c\\5_Cooling_2nd_try\\September_2014\\091814\\14.37100K_500_2500_2.10000V_0.00000T_Sep18-2014__03-25-07_001_091814.bin", "mod time(min)"=58231165.11666667, "file format"=enum."binary", "power(V)"=2.1, "Magn Field(T) "=0.0}, {"temperature"=14.369, "temperature str"="14.36900", "file path"=path "D:/Data/Ultrasound/LSCO/LSCO22__130814c/5_Cooling_2nd_try/September_2014/091814/14.36900K_500_2500_2.10000V_0.00000T_Sep18-2014__03-26-27_001_091814.bin", "last mod"=timestamp(3493869987 s since 1904-01-01), "file name str"="D:\\Data\\Ultrasound\\LSCO\\LSCO22__130814c\\5_Cooling_2nd_try\\September_2014\\091814\\14.36900K_500_2500_2.10000V_0.00000T_Sep18-2014__03-26-27_001_091814.bin", "mod time(min)"=58231166.45, "file format"=enum."binary", "power(V)"=2.1, "Magn Field(T) "=0.0}, {"temperature"=14.369, "temperature str"="14.36900", "file path"=path "D:/Data/Ultrasound/LSCO/LSCO22__130814c/5_Cooling_2nd_try/September_2014/091814/14.36900K_500_2500_2.10000V_0.00000T_Sep18-2014__03-27-46_001_091814.bin", "last mod"=timestamp(3493870066 s since 1904-01-01), "file name str"="D:\\Data\\Ultrasound\\LSCO\\LSCO22__130814c\\5_Cooling_2nd_try\\September_2014\\091814\\14.36900K_500_2500_2.10000V_0.00000T_Sep18-2014__03-27-46_001_091814.bin", "mod time(min)"=58231167.766666666, "file format"=enum."binary", "power(V)"=2.1, "Magn Field(T) "=0.0}, {"temperature"=14.373, "temperature str"="14.37300", "file path"=path "D:/Data/Ultrasound/LSCO/LSCO22__130814c/5_Cooling_2nd_try/September_2014/091814/14.37300K_500_2500_2.10000V_0.00000T_Sep18-2014__03-29-06_001_091814.bin", "last mod"=timestamp(3493870146 s since 1904-01-01), "file name str"="D:\\Data\\Ultrasound\\LSCO\\LSCO22__130814c\\5_Cooling_2nd_try\\September_2014\\091814\\14.37300K_500_2500_2.10000V_0.00000T_Sep18-2014__03-29-06_001_091814.bin", "mod time(min)"=58231169.1, "file format"=enum."binary", "power(V)"=2.1, "Magn Field(T) "=0.0}, {"temperature"=14.37, "temperature str"="14.37000", "file path"=path "D:/Data/Ultrasound/LSCO/LSCO22__130814c/5_Cooling_2nd_try/September_2014/091814/14.37000K_500_2500_2.10000V_0.00000T_Sep18-2014__03-30-25_001_091814.bin", "last mod"=timestamp(3493870225 s since 1904-01-01), "file name str"="D:\\Data\\Ultrasound\\LSCO\\LSCO22__130814c\\5_Cooling_2nd_try\\September_2014\\091814\\14.37000K_500_2500_2.10000V_0.00000T_Sep18-2014__03-30-25_001_091814.bin", "mod time(min)"=58231170.416666664, "file format"=enum."binary", "power(V)"=2.1, "Magn Field(T) "=0.0}, {"temperature"=14.368, "temperature str"="14.36800", "file path"=path "D:/Data/Ultrasound/LSCO/LSCO22__130814c/5_Cooling_2nd_try/September_2014/091814/14.36800K_500_2500_2.10000V_0.00000T_Sep18-2014__03-31-44_001_091814.bin", "last mod"=timestamp(3493870304 s since 1904-01-01), "file name str"="D:\\Data\\Ultrasound\\LSCO\\LSCO22__130814c\\5_Cooling_2nd_try\\September_2014\\091814\\14.36800K_500_2500_2.10000V_0.00000T_Sep18-2014__03-31-44_001_091814.bin", "mod time(min)"=58231171.733333334, "file format"=enum."binary", "power(V)"=2.1, "Magn Field(T) "=0.0}, {"temperature"=14.366, "temperature str"="14.36600", "file path"=path "D:/Data/Ultrasound/LSCO/LSCO22__130814c/5_Cooling_2nd_try/September_2014/091814/14.36600K_500_2500_2.10000V_0.00000T_Sep18-2014__03-33-04_001_091814.bin", "last mod"=timestamp(3493870384 s since 1904-01-01), "file name str"="D:\\Data\\Ultrasound\\LSCO\\LSCO22__130814c\\5_Cooling_2nd_try\\September_2014\\091814\\14.36600K_500_2500_2.10000V_0.00000T_Sep18-2014__03-33-04_001_091814.bin", "mod time(min)"=58231173.06666667, "file format"=enum."binary", "power(V)"=2.1, "Magn Field(T) "=0.0}, {"temperature"=14.363, "temperature str"="14.36300", "file path"=path "D:/Data/Ultrasound/LSCO/LSCO22__130814c/5_Cooling_2nd_try/September_2014/091814/14.36300K_500_2500_2.10000V_0.00000T_Sep18-2014__03-34-23_001_091814.bin", "last mod"=timestamp(3493870463 s since 1904-01-01), "file name str"="D:\\Data\\Ultrasound\\LSCO\\LSCO22__130814c\\5_Cooling_2nd_try\\September_2014\\091814\\14.36300K_500_2500_2.10000V_0.00000T_Sep18-2014__03-34-23_001_091814.bin", "mod time(min)"=58231174.38333333, "file format"=enum."binary", "power(V)"=2.1, "Magn Field(T) "=0.0}, {"temperature"=14.364, "temperature str"="14.36400", "file path"=path "D:/Data/Ultrasound/LSCO/LSCO22__130814c/5_Cooling_2nd_try/September_2014/091814/14.36400K_500_2500_2.10000V_0.00000T_Sep18-2014__03-35-43_001_091814.bin", "last mod"=timestamp(3493870543 s since 1904-01-01), "file name str"="D:\\Data\\Ultrasound\\LSCO\\LSCO22__130814c\\5_Cooling_2nd_try\\September_2014\\091814\\14.36400K_500_2500_2.10000V_0.00000T_Sep18-2014__03-35-43_001_091814.bin", "mod time(min)"=58231175.71666667, "file format"=enum."binary", "power(V)"=2.1, "Magn Field(T) "=0.0}, {"temperature"=14.367, "temperature str"="14.36700", "file path"=path "D:/Data/Ultrasound/LSCO/LSCO22__130814c/5_Cooling_2nd_try/September_2014/091814/14.36700K_500_2500_2.10000V_0.00000T_Sep18-2014__03-37-02_001_091814.bin", "last mod"=timestamp(3493870622 s since 1904-01-01), "file name str"="D:\\Data\\Ultrasound\\LSCO\\LSCO22__130814c\\5_Cooling_2nd_try\\September_2014\\091814\\14.36700K_500_2500_2.10000V_0.00000T_Sep18-2014__03-37-02_001_091814.bin", "mod time(min)"=58231177.03333333, "file format"=enum."binary", "power(V)"=2.1, "Magn Field(T) "=0.0}, {"temperature"=14.363, "temperature str"="14.36300", "file path"=path "D:/Data/Ultrasound/LSCO/LSCO22__130814c/5_Cooling_2nd_try/September_2014/091814/14.36300K_500_2500_2.10000V_0.00000T_Sep18-2014__03-38-21_001_091814.bin", "last mod"=timestamp(3493870701 s since 1904-01-01), "file name str"="D:\\Data\\Ultrasound\\LSCO\\LSCO22__130814c\\5_Cooling_2nd_try\\September_2014\\091814\\14.36300K_500_2500_2.10000V_0.00000T_Sep18-2014__03-38-21_001_091814.bin", "mod time(min)"=58231178.35, "file format"=enum."binary", "power(V)"=2.1, "Magn Field(T) "=0.0}, {"temperature"=14.363, "temperature str"="14.36300", "file path"=path "D:/Data/Ultrasound/LSCO/LSCO22__130814c/5_Cooling_2nd_try/September_2014/091814/14.36300K_500_2500_2.10000V_0.00000T_Sep18-2014__03-39-41_001_091814.bin", "last mod"=timestamp(3493870781 s since 1904-01-01), "file name str"="D:\\Data\\Ultrasound\\LSCO\\LSCO22__
